vi "DAQ.Channels.Override.vi"(8 "error in (no error)":errorcluster, 10 "DAQ.Channels":T1, 11 "DAQ in":refnum<class "DAQ.lvclass">) -> (0 "error out":errorcluster, 3 "DAQ out":refnum<class "DAQ.lvclass">)   [LabVIEW 2016, in "DAQ.lvclass"]
uses:
  DAQ.lvclass
  Typedefs/PublicEvents--DAQ.Channels.ctl
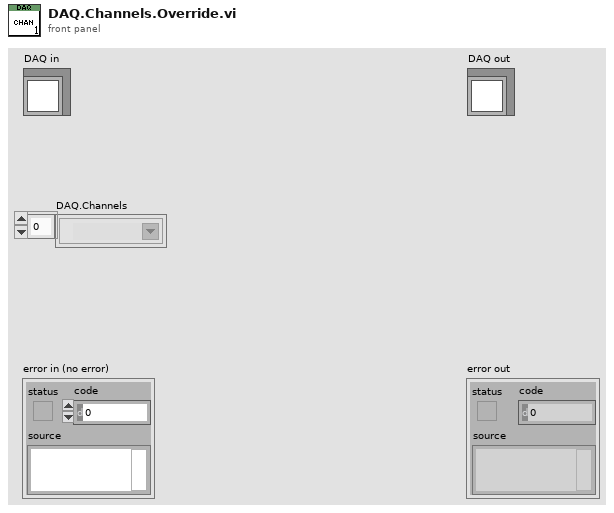
[diagram p1: front panel]
types:
  T1 = typedef "DAQ.lvclass/PublicEvents--DAQ.Channels.ctl" = tag[]
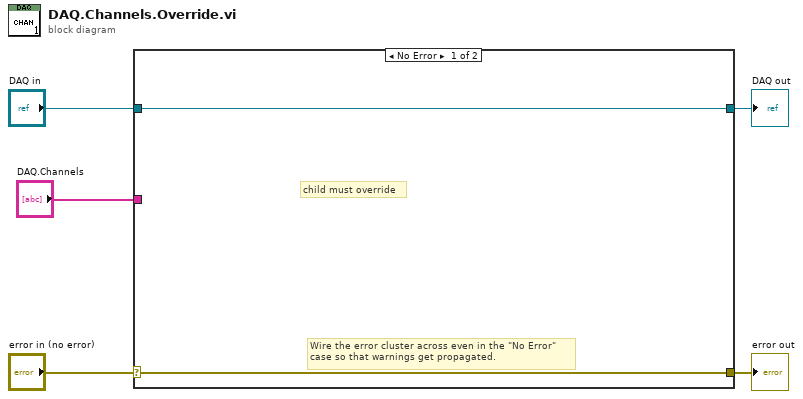
[diagram p0: block diagram]
diagram:
  n1 = case shown="No Error" "error in (no error)" {
    selector: "error in (no error)" -> [w6 w9]
    tunnel: [w6 w9] -> w4
    tunnel: [w7 w8] -> w2
    tunnel: "DAQ in" -> [w7 w8]
    tunnel: "DAQ.Channels" -> [_ _]
    frame No Error {
      # "child must override"
      # "Wire the error cluster across even in the \"No Error\"\ncase so that warnings get propagated."
    }
    frame Error {
    }
  }
  "error out" <- w4
  "DAQ out" <- w2
